vi "getRanges.vi"(0 "AnalogOutput.lvclass in":refnum<class "AnalogOutput.lvclass">, 1 "error in (no error)":errorcluster) -> (2 "AnalogOutput.lvclass out":refnum<class "AnalogOutput.lvclass">, 3 "Ranges":dbl[](array[numeric]), 4 "error out":errorcluster)   [LabVIEW 2009, in "Hardware.lvlib" / "Channels.lvlib" / "AnalogOutput.lvclass"]
uses:
  AnalogOutput.lvclass
  AnalogOutput.lvclass/AnalogOutput.ctl
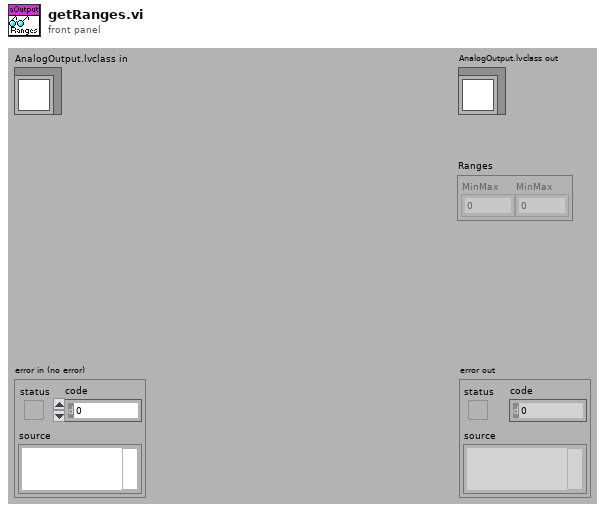
[diagram p1: front panel]
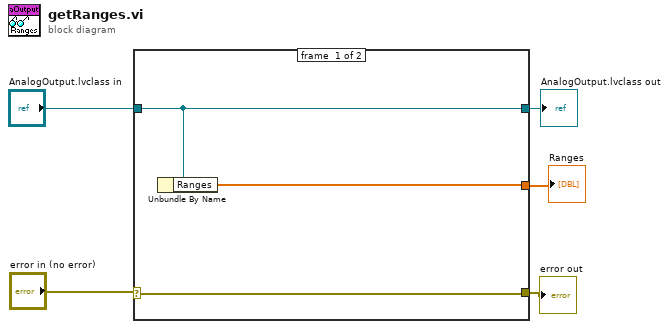
[diagram p0: block diagram]
diagram:
  n1 = case shown="No Error" "error in (no error)" {
    selector: "error in (no error)" -> [w8 w9]
    tunnel: [w8 w9] -> w4
    tunnel: [w7 w10] -> w2
    tunnel: "AnalogOutput.lvclass in" -> [w7 w10]
    tunnel: [w6 _] -> w1
    frame #0 {
      n2 = Unbundle By Name(w7) -> ("Ranges"=w6:dbl[])
    }
    frame #1 {
    }
  }
  "error out" <- w4
  "AnalogOutput.lvclass out" <- w2
  "Ranges" <- w1
